vi "Label Targets Ball.vi"(5 "Details":bool, 7 "Annotate":bool=TRUE, 8 "Score Threshold":dbl, 9 "results":T1, 11 "Image in":T2) -> (3 "Image out":T2)   [LabVIEW 2019]
doc: "Draw scores near or on the particle and an ellipse around the target. Scores that are below the score threshold are drawn in red, above in green."
uses:
  <vilib>/vision/Image Controls.llb/IMAQ Image.ctl
  Vision Support Code/Target Fields.ctl
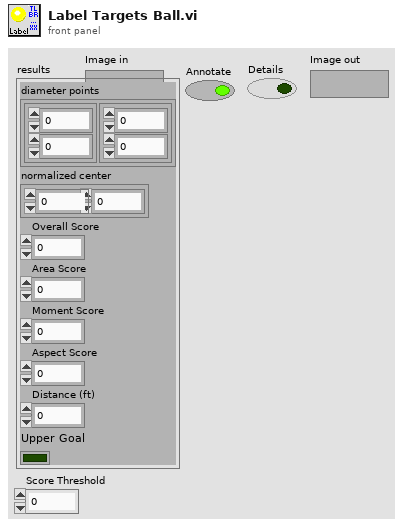
[diagram p1: front panel]
types:
  T1 = typedef "Target Fields.ctl" = cluster{"diameter points":cluster{"first point":cluster{"x":dbl, "y":dbl}, "projected point":cluster{"x":dbl, "y":dbl}}, "normalized center":cluster{"x":dbl, "y":dbl}, "Overall Score":dbl, "Area Score":dbl, "Moment Score":dbl, "Aspect Score":dbl, "Distance (ft)":dbl, "Upper Goal":bool}
  T2 = typedef "IMAQ Image.ctl" = refnum<image>
  T3 = cluster{"Desired Font (Application)":enum16{"User-specified Font", "Application Font", "System Font", "Dialog Font"}, "[User-specified Font]":cluster{"Font Name":string, "Size":i16, "Strikeout?":bool, "Italic?":bool, "Underline?":bool, "Outline?":bool, "Shadow?":bool, "Bold?":bool, "Rotation Angle":dbl}, "Horizontal Alignment":i16, "Vertical Alignment":i16}
  T4 = cluster{"first point":cluster{"x":dbl, "y":dbl}, "projected point":cluster{"x":dbl, "y":dbl}}
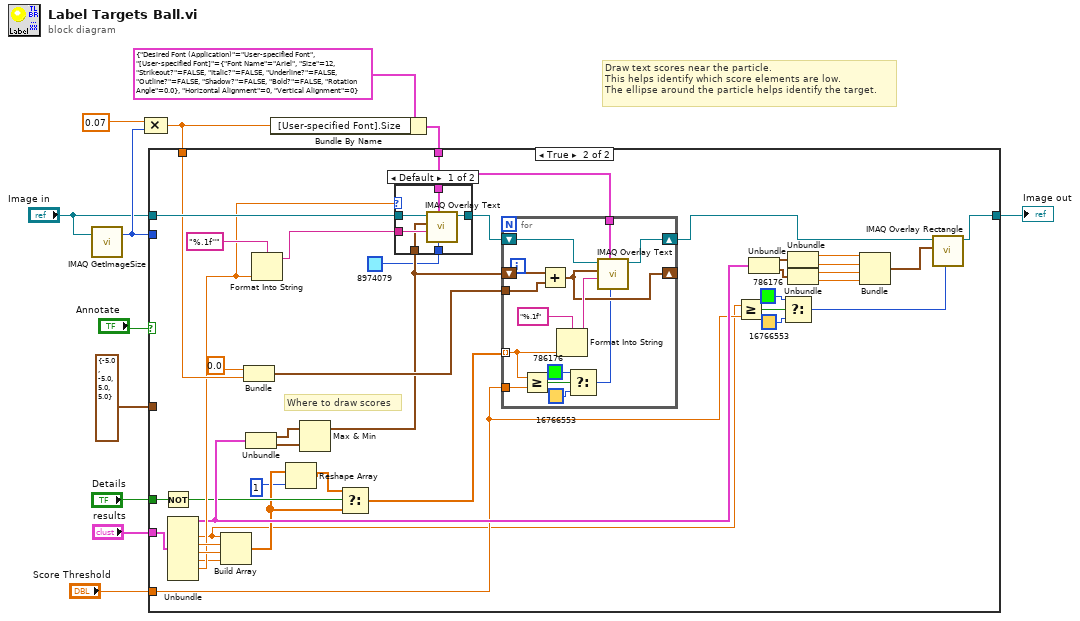
[diagram p0: block diagram]
diagram:
  # "Draw text scores near the particle.\nThis helps identify which score elements are low.\nThe ellipse around the particle helps identify the target."
  n1 = call "IMAQ GetImageSize"("Image"="Image in") -> ("Y Resolution"=w9:i32)  [unwired: 3 in, 2 out]
  n2 = Compound Arithmetic op=MULTIPLY(0.07, w9) -> (w5:dbl)
  n3 = Bundle By Name(cluster=T3 {"Desired Font (Application)"=enum."User-specified Font", "[User-specified Font]"={"Font Name"="Ariel", "Size"=12, "Strikeout?"=FALSE, "Italic?"=FALSE, "Underline?"=FALSE, "Outline?"=FALSE, "Shadow?"=FALSE, "Bold?"=FALSE, "Rotation Angle"=0.0}, "Horizontal Alignment"=0, "Vertical Alignment"=0} ("Font, Size & Style"), "[User-specified Font].Size"=w5) -> (w6:T3)
  n4 = case shown="True" "Annotate" {
    tunnel: [w13 w46] -> w12
    tunnel: "Image in" -> [w13 w52]
    tunnel: w6 -> [_ w34]
    tunnel: w9 -> [_ _]
    tunnel: cluster{dbl, dbl, dbl, dbl} {-5.0, -5.0, 5.0, 5.0} ("output cluster") -> [_ _]
    tunnel: w5 -> [_ w48]
    tunnel: "results" -> [_ w47]
    tunnel: "Score Threshold" -> [_ w15]
    tunnel: "Details" -> [_ w25]
    frame False {
    }
    frame True {
      # "Where to draw scores"
      n5 = Not(x=w25) -> (.not. x?=w24:bool)
      n6 = Unbundle(w47) -> ("diameter points"=w33:T4, "Overall Score"=w14:dbl, "Area Score"=w45:dbl, "Moment Score"=w38:dbl, "Aspect Score"=w35:dbl, "Distance (ft)"=w36:dbl)  [unwired: 2 out]
      n7 = Build Array(w14, w45, w38, w35) -> (w22:dbl[])
      n8 = Bundle(0.0, w48) -> (w42:cluster{dbl, dbl})  [unwired: 1 in]
      n9 = Unbundle(w33) -> ("first point"=w40:cluster{"x":dbl, "y":dbl}, "projected point"=w41:cluster{"x":dbl, "y":dbl})
      n10 = Format Into String(format string="%.1f''", w36) -> (resulting string=w51:string)  [unwired: 2 in, 1 out]
      n11 = Reshape Array(w22, 1) -> (w23:dbl[])
      n12 = Max & Min(x=w40, y=w41) -> (max(x,y)=w39:cluster{"x":dbl, "y":dbl})  [unwired: 1 out]
      n13 = Select(t=w23, s=w24, f=w22) -> (s? t:f=w21:dbl[])
      n14 = case shown="Default" w36 {
        tunnel: w52 -> [w72 w73]
        tunnel: w51 -> [w71 _]
        tunnel: w34 -> [w70 _]
        tunnel: [w69 w73] -> w44
        tunnel: w39 -> [w68 _]
        tunnel: u32 8974079 ("Color") -> [w67 _]
        frame Default {
          n15 = call "IMAQ Overlay Text"("Text Color (black)"=w67, "Font, Size & Style"=w70, "String"=w71, "Origin"=w68, "Image"=w72) -> ("Image Out"=w69:T2)  [unwired: 5 in, 1 out]
        }
        frame 0 {
        }
      }
      n16 = for {
        tunnel: w21 -> [w55] mode=indexing
        shift-right: [w63] -> w43
        shift-left: w44 -> [w64]
        tunnel: w34 -> [w62]
        shift-right: [w59] -> _
        shift-left: w39 -> [w60]
        tunnel: w42 -> [w61]
        tunnel: w15 -> [w54]
        n17 = Greater Or Equal?(x=w55, y=w54) -> (x >= y?=w53:bool)
        n18 = Add(x=w60, y=w61) -> (x+y=w59:cluster{dbl, dbl})
        n19 = Format Into String(format string="%.1f", w55) -> (resulting string=w65:string)  [unwired: 2 in, 1 out]
        n20 = Select(t=u32 786176 ("Color"), s=w53, f=u32 16766553 ("Color")) -> (s? t:f=w56:u32)
        n21 = call "IMAQ Overlay Text"("Text Color (black)"=w56, "Font, Size & Style"=w62, "String"=w65, "Origin"=w59, "Image"=w64) -> ("Image Out"=w63:T2)  [unwired: 5 in, 1 out]
      }
      n22 = Greater Or Equal?(x=w14, y=w15) -> (x >= y?=w16:bool)
      n23 = Unbundle(w33) -> ("first point"=w32:cluster{"x":dbl, "y":dbl}, "projected point"=w31:cluster{"x":dbl, "y":dbl})
      n24 = Select(t=u32 786176 ("Color"), s=w16, f=u32 16766553 ("Color")) -> (s? t:f=w17:u32)
      n25 = Unbundle(w32) -> ("x"=w30:dbl, "y"=w29:dbl)
      n26 = Unbundle(w31) -> ("x"=w28:dbl, "y"=w27:dbl)
      n27 = Bundle("x"=w30, "y"=w29, "x"=w28, "y"=w27) -> (w26:cluster{"x":dbl, "y":dbl, "x":dbl, "y":dbl})  [unwired: 1 in]
      n28 = call "IMAQ Overlay Rectangle"("Color"=w17, "Rectangle"=w26, "Image"=w43) -> ("Image Out"=w46:T2)  [unwired: 7 in, 1 out]
    }
  }
  "Image out" <- w12
